vi "i2c bus monitor.vi"() -> ()   [LabVIEW 2025]
uses:
  <vilib>/userDefined/Silver/nirio_resource_slv.ctl
panel:
  out "RIO Device 2":T1="PXI1Slot8"
  in  "error in (no error)":errorcluster
  out "Bitfile Path":path
  in  "RIO Device":T1="PXI1Slot8"
  out "Serial Input Channels":string[](array[string])
  out "SI Count":i32
  out "Module Name":string
  out "error out":errorcluster
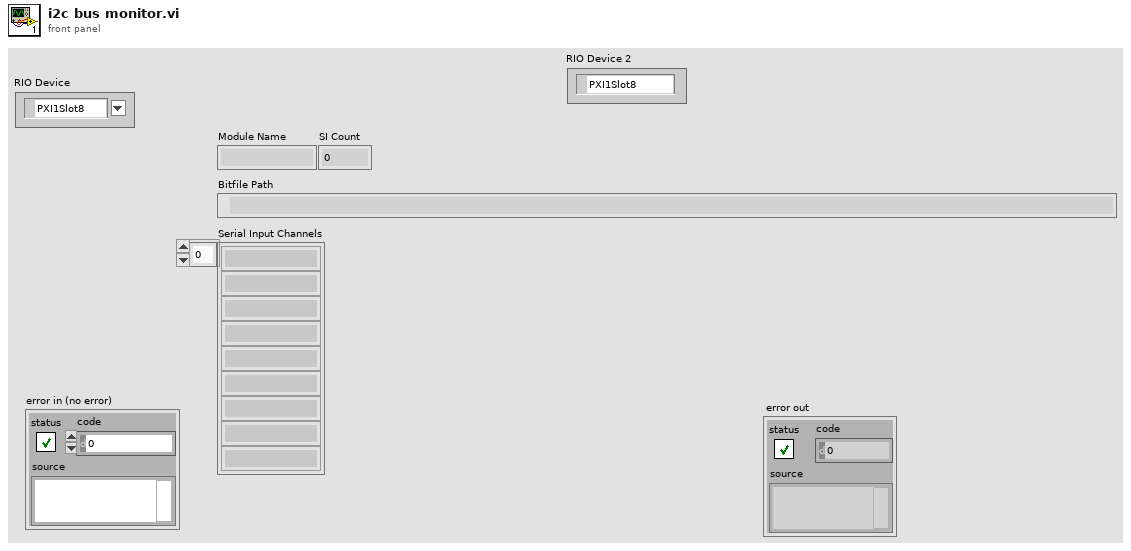
[diagram p1: front panel]
types:
  T1 = typedef "nirio_resource_slv.ctl" = tag
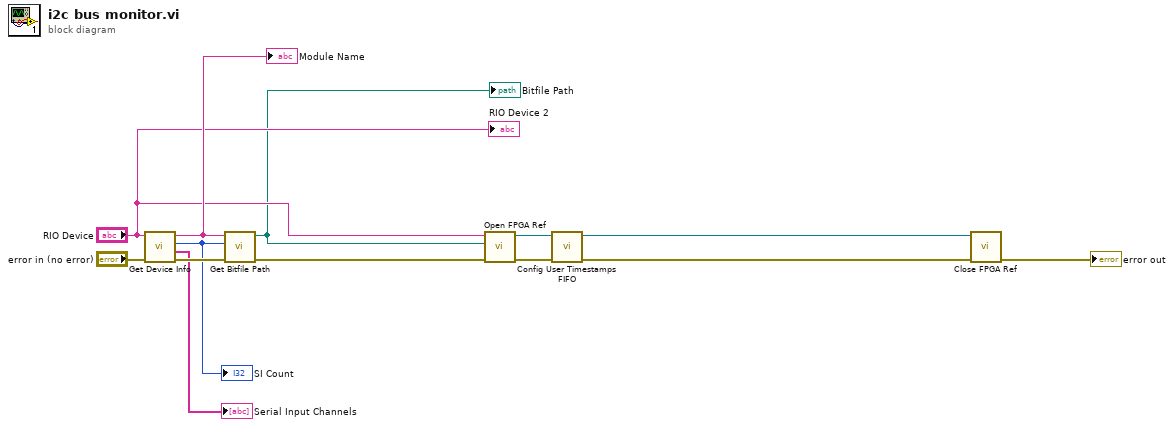
[diagram p0: block diagram]
diagram:
  n1 = call "Get Device Info.vi"("error in (no error)"="error in (no error)", "RIO Device"="RIO Device") -> ("error out"=w13:errorcluster, "SI Channels"=→"Serial Input Channels":string[], "SI Count"=w10:i32, "Module Name"=w9:string)  [unwired: 6 in]
  "Module Name" <- w9
  "SI Count" <- w10
  n2 = call "Get Bitfile Path.vi"("error in (no error)"=w13, "SI Count"=w10, "Module Name"=w9) -> ("error out"=w8:errorcluster, "Bitfile Path"=w5:path)  [unwired: 7 in]
  "Bitfile Path" <- w5
  n3 = call "Open FPGA Ref.vi"("error in (no error)"=w8, "Bitfile Path"=w5, "Device address"="RIO Device") -> ("error out"=w3:errorcluster, "FPGA Ref out"=w4:refnum<k20>)  [unwired: 7 in]
  n4 = call "Config User Timestamps FIFO.vi"("error in (no error)"=w3, "FPGA Ref in"=w4) -> ("error out"=w1:errorcluster, "FPGA Ref out"=w2:refnum<k20>)  [unwired: 8 in]
  n5 = call "Close FPGA Ref.vi"("error in (no error)"=w1, "FPGA Ref in"=w2) -> ("error out"=→"error out":errorcluster)  [unwired: 9 in]
  "RIO Device 2" <- "RIO Device"
